vi "VISA RW.vi"(8 "error in (no error)":errorcluster, 10 "Write":string, 11 "VISA Refnum in":refnum<visa-resource-name>) -> (0 "error out":errorcluster, 2 "Read":string, 3 "VISA Refnum out":refnum<visa-resource-name>)   [LabVIEW 2019, in "RP100.lvlib"]
uses:
  RP100.lvlib
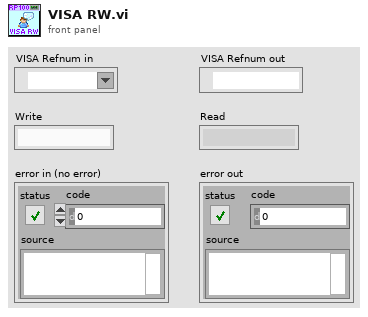
[diagram p1: front panel]
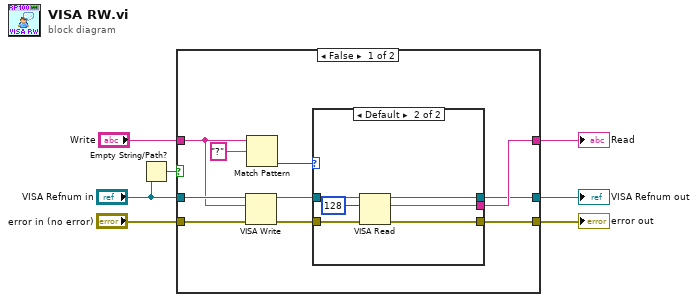
[diagram p0: block diagram]
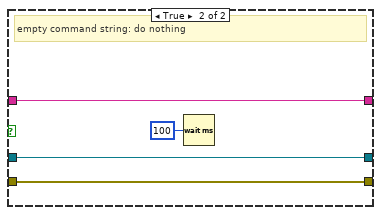
[diagram p3: hidden frame]
diagram:
  n1 = Empty String/Path?(string/path="VISA Refnum in") -> (empty?=w2:bool)
  n2 = case shown="False" w2 {
    tunnel: "error in (no error)" -> [w17 w27]
    tunnel: [w16 w29] -> w6
    tunnel: [w15 w27] -> w5
    tunnel: "VISA Refnum in" -> [w14 w28]
    tunnel: [w13 w28] -> w4
    tunnel: "Write" -> [w12 w29]
    frame False {
      n3 = VISA Write(VISA resource name=w14, write buffer=w12, error in (no error)=w17) -> (VISA resource name out=w9:refnum<visa-resource-name>, error out=w10:errorcluster)  [unwired: 1 out]
      n4 = Match Pattern(string=w12, regular expression="?") -> (offset past match=w8:i32)  [unwired: 1 in, 3 out]
      n5 = case shown="Default" w8 {
        tunnel: [_ w25] -> w16
        tunnel: [w18 w24] -> w15
        tunnel: [w19 w23] -> w13
        tunnel: w10 -> [w18 w22]
        tunnel: w9 -> [w19 w21]
        frame -1 {
          # "-1: no \"?\" match, do not read buffer"
        }
        frame Default {
          n6 = VISA Read(VISA resource name=w21, byte count=u32 128, error in (no error)=w22) -> (VISA resource name out=w23:refnum<visa-resource-name>, read buffer=w25:string, error out=w24:errorcluster)  [unwired: 1 out]
        }
      }
    }
    frame True {
      # "empty command string: do nothing"
      n7 = Wait (ms)(milliseconds to wait=u32 100) -> ()  [unwired: 1 out]
    }
  }
  "Read" <- w6
  "error out" <- w5
  "VISA Refnum out" <- w4
